vi "daq1.vi"() -> ()   [LabVIEW 2011]
panel:
  in  "llenar":i32(knob) scale=0.0..5.0
  out "tanque":dbl(slide) scale=0.0..10.0
  out "foco":bool
  in  "on/off":bool
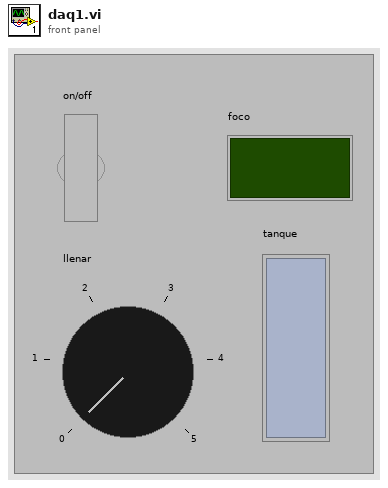
[diagram p1: front panel]
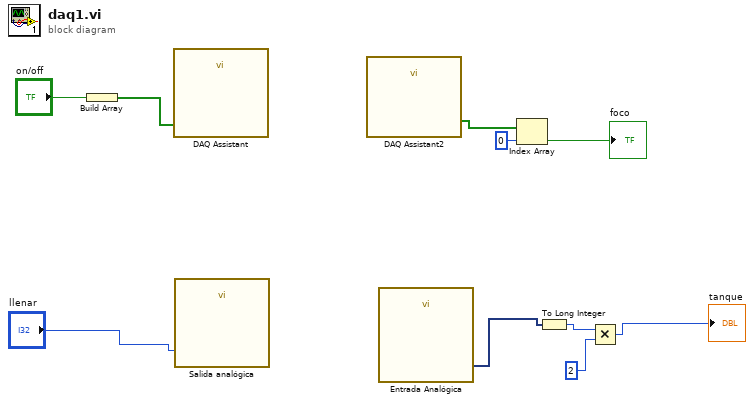
[diagram p0: block diagram]
diagram:
  n1 = Build Array "Build Array"("on/off") -> (w4:bool[])
  n2 = call "DAQ Assistant"("data"=w4) -> ()  [unwired: 17 in, 2 out]
  n3 = call "Salida analógica"("data"="llenar") -> ()  [unwired: 17 in, 2 out]
  n4 = call "DAQ Assistant2"() -> ("data"=w3:bool[])  [unwired: 17 in, 2 out]
  n5 = call "Entrada Analógica"() -> ("data"=w6:dynamicdata)  [unwired: 17 in, 2 out]
  n6 = Index Array "Index Array"(array=w3, index=0) -> (element=→"foco":bool)
  n7 = To Long Integer(number=w6) -> (32bit integer=w10:i32)
  n8 = Multiply(x=w10, y=2) -> (x*y=→"tanque":i32)
